vi "Log battery data to TDMS.vi"(4 "TDMS File Path In":string, 6 "Current (mA)":dbl[](array[numeric]), 7 "Cycle":i32, 9 "Voltage (V)":dbl[](array[numeric]), 10 "Energy (Wh)":dbl, 11 "Capacity  (mAh)":dbl) -> (3 "TDMS File Path Out":string)   [LabVIEW 2019]
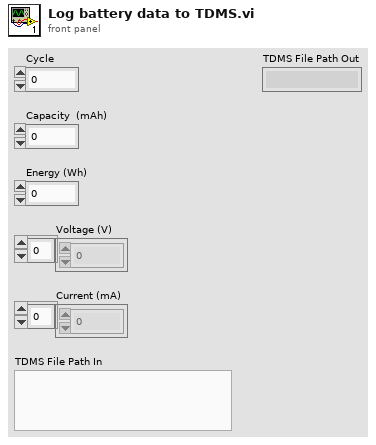
[diagram p1: front panel]
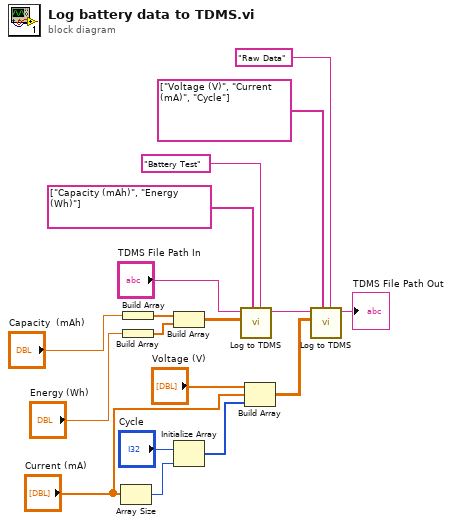
[diagram p0: block diagram]
diagram:
  n1 = Array Size(array="Current (mA)") -> (size(s)=w17:i32)
  n2 = Build Array("Capacity  (mAh)") -> (w4:dbl[])
  n3 = Build Array("Energy (Wh)") -> (w5:dbl[])
  n4 = Build Array(w4, w5) -> (w9:dbl[][])
  n5 = Initialize Array("Cycle", w17) -> (w16:i32[])
  n6 = call "Log to TDMS.vi"("group name in (Untitled)"="Battery Test", "channel name(s) in (Untitled)"=string[] ["Capacity (mAh)", "Energy (Wh)"], "Array"=w9, "TDMS File Path In"="TDMS File Path In") -> ("String"=w10:string)  [unwired: 7 in]
  n7 = Build Array("Voltage (V)", "Current (mA)", w16) -> (w12:dbl[][])
  n8 = call "Log to TDMS.vi"("group name in (Untitled)"="Raw Data", "channel name(s) in (Untitled)"=string[] ["Voltage (V)", "Current (mA)", "Cycle"], "Array"=w12, "TDMS File Path In"=w10) -> ("String"=→"TDMS File Path Out":string)  [unwired: 7 in]
